vi "Generate trace XY.vi"(9 "Density":dbl=1.275, 10 "Blade Lenth":dbl=40.0, 11 "Windspeeds":dbl[][](array[numeric])) -> (2 "Trace Y":dbl[][](array[numeric]), 3 "Trace X":dbl[][](array[numeric]))   [LabVIEW 2009]
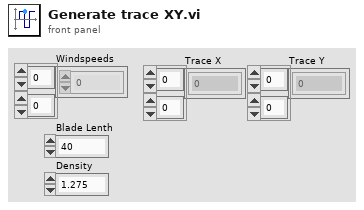
[diagram p1: front panel]
types:
  T1 = cluster{"Name":string, "Color":u32, "Style":u8, "Point Style":u8, "Name Visible":bool, "Allow Drag":bool, "Annotation Mode":u32, "Plot":i32, "Index":i32, "Position":cluster{"X":dbl, "Y":dbl}, "X Scale":u32, "Y Scale":u32, "Show Arrow":bool, "Lock Name":bool, "Plot Area":i32, "Label Offset":cluster{"X":dbl, "Y":dbl}}
  T2 = cluster{"Name":string, "Color":u32, "Style":u8, "Point Style":u8, "Name Visible":bool, "Allow Drag":bool, "Annotation Mode":u32, "Plot":i32, "Index":i32, "Position":cluster{"X":dbl, "Y":dbl}, "X Scale":u32, "Y Scale":u32, "Show Arrow":bool, "Lock Name":bool, "Plot Area":i32, "Label Offset":cluster{"X":dbl, "Y":dbl}}[]
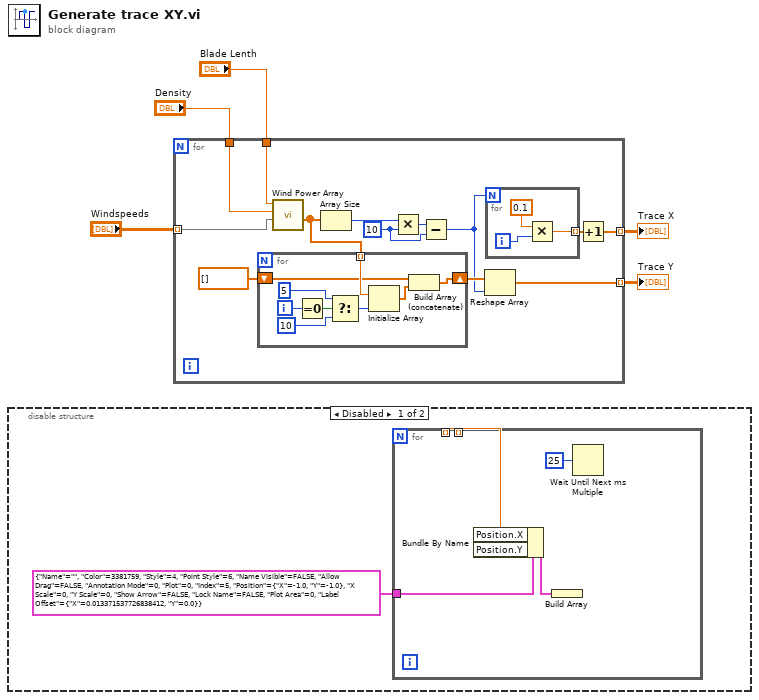
[diagram p0: block diagram]
diagram:
  n1 = disable-structure shown="Disabled" {
    frame #0 {
      n2 = for {
        tunnel: T1 {"Name"="", "Color"=3381759, "Style"=4, "Point Style"=6, "Name Visible"=FALSE, "Allow Drag"=FALSE, "Annotation Mode"=0, "Plot"=0, "Index"=5, "Position"={"X"=-1.0, "Y"=-1.0}, "X Scale"=0, "Y Scale"=0, "Show Arrow"=FALSE, "Lock Name"=FALSE, "Plot Area"=0, "Label Offset"={"X"=0.013371537726838412, "Y"=0.0}} -> [w10]
        tunnel: _ -> [w7] mode=indexing
        tunnel: _ -> [w8] mode=indexing
        n3 = Bundle By Name(cluster=w10, "Position.X"=w8, "Position.Y"=w7) -> (w9:T1)
        n4 = Build Array(w9) -> (w12:T2)
        n5 = Wait Until Next ms Multiple(millisecond multiple=u32 25) -> ()  [unwired: 1 out]
      }
    }
    frame #1 {
    }
  }
  n6 = for {
    tunnel: [w19] -> w5 mode=indexing
    tunnel: [w17] -> w4 mode=indexing
    tunnel: "Windspeeds" -> [w15] mode=indexing
    tunnel: "Blade Lenth" -> [w14]
    tunnel: "Density" -> [w13]
    w22 = 10 ("y")
    n7 = call "Wind Power Array.vi"("Wind Speed (m/s)"=w15, "Density (kg/m^3)"=w13, "Blade Length (m)"=w14) -> ("Power (watts)"=w16:dbl[])  [unwired: 8 in]
    n8 = for {
      tunnel: w16 -> [w37] mode=indexing
      shift-right: [w29] -> w21
      shift-left: dbl[] [] -> [w30]
      i -> [w36]
      n9 = Equal To 0?(x=w36) -> (x = 0?=w35:bool)
      n10 = Select(t=5 ("dimension size"), s=w35, f=10 ("dimension size")) -> (s? t:f=w32:i32)
      n11 = Initialize Array(w37, w32) -> (w31:dbl[])
      n12 = Build Array (concatenate)(w30, w31) -> (w29:dbl[])
    }
    n13 = Array Size(array=w16) -> (size(s)=w24:i32)
    n14 = Multiply(x=w24, y=w22) -> (x*y=w23:i32)
    n15 = Subtract(x=w23, y=w22) -> (x-y=w20:i32)
    n16 = Reshape Array(w21, w20) -> (w19:dbl[])
    n17 = for {
      N: w20 -> [_]
      tunnel: [w26] -> w18 mode=indexing
      i -> [w28]
      n18 = Multiply(x=0.1, y=w28) -> (x*y=w26:dbl)
    }
    n19 = Increment(x=w18) -> (x+1=w17:dbl[])
  }
  "Trace X" <- w4
  "Trace Y" <- w5
